vi "autoconfigure devices and accesspoint wireless.vi"(10 "wireless_channel_number":u8, 11 "context":u32) -> (2 "function return":i32, 3 "context out":u32)   [LabVIEW 2019, in "apdm.lvlib"]
doc: "APDM_EXPORT int apdm_autoconfigure_devices_and_accesspoint_wireless(apdm_ctx_t context, const uint8_t wireless_channel_number);"
uses:
  apdm.lvlib
  Lee Lab/CP FES Walking 2018/Code/Working/LabVIEW/apdm.dll
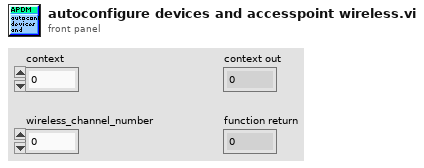
[diagram p1: front panel]
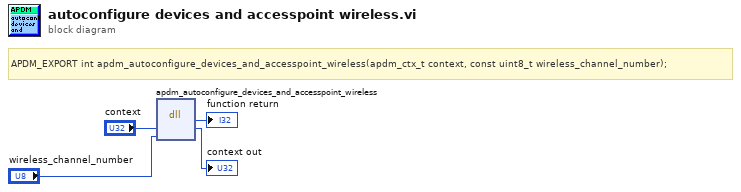
[diagram p0: block diagram]
diagram:
  # "APDM_EXPORT int apdm_autoconfigure_devices_and_accesspoint_wireless(apdm_ctx_t context, const uint8_t wireless_channel_number);"
  n1 = dll-call lib="C:/Users/jfalesi/Dropbox/Lee Lab/CP FES Walking 2018/Code/Working/LabVIEW/apdm.*" fn="apdm_autoconfigure_devices_and_accesspoint_wireless"("context"="context", "wireless_channel_number"="wireless_channel_number") -> (→"function return":i32, "context"=→"context out":u32)  [unwired: 4 in, 2 out]
